vi "VG_ALIM.vi"() -> ()   [LabVIEW 2020]
panel:
  out "ALIM":string
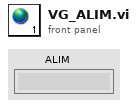
[diagram p1: front panel]
diagram:
